vi "CFTS-Get Data Folder.vi"(5 "Drive":string, 7 "Root folder":path, 8 "error in (no error)":errorcluster, 9 "create?":bool, 10 "Number":i32, 11 "Experimenter":string) -> (0 "error out":errorcluster, 2 "Data folder":path)   [LabVIEW 2020]
doc: "Takes an experiment ID (e.g. KEH999) and returns the standard data folder (e.g. C:\\Data\\KEH DATA\\KEH999)"
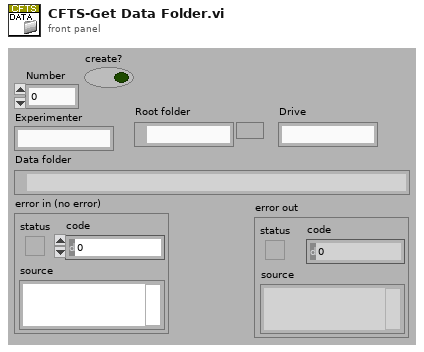
[diagram p1: front panel]
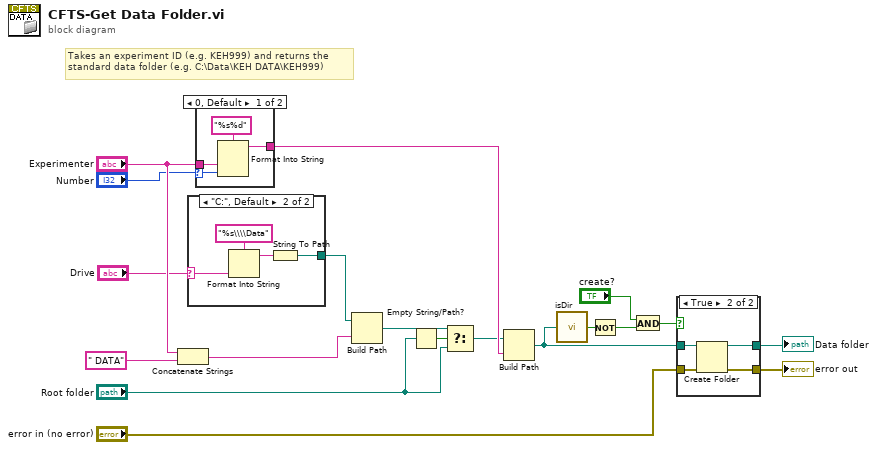
[diagram p0: block diagram]
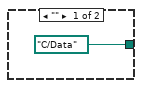
[diagram p2: hidden frame]
diagram:
  # "Takes an experiment ID (e.g. KEH999) and returns the\nstandard data folder (e.g. C:\\Data\\KEH DATA\\KEH999)"
  n1 = Concatenate Strings("Experimenter", " DATA" ("string")) -> (w18:string)
  n2 = case shown="\"C:\", Default" "Drive" {
    selector: "Drive" -> [_ w23]
    tunnel: [path "C:/Data" ("base path") w21] -> w1
    frame "" {
    }
    frame "C:", Default {
      n3 = Format Into String(format string="%s\\\\Data", w23) -> (resulting string=w22:string)  [unwired: 2 in, 1 out]
      n4 = String To Path(string=w22) -> (path=w21:path)
    }
  }
  n5 = case shown="0, Default" "Number" {
    selector: "Number" -> [w26 _]
    tunnel: "Experimenter" -> [w27 w29]
    tunnel: [w25 w29] -> w15
    frame 0, Default {
      n6 = Format Into String(format string="%s%d", w27, w26) -> (resulting string=w25:string)  [unwired: 2 in, 1 out]
    }
    frame -1 {
    }
  }
  n7 = Build Path(base path=w1, name or relative path=w18) -> (appended path=w5:path)
  n8 = Empty String/Path?(string/path="Root folder") -> (empty?=w6:bool)
  n9 = Select(t=w5, s=w6, f="Root folder") -> (s? t:f=w4:path)
  n10 = Build Path(base path=w4, name or relative path=w15) -> (appended path=w14:path)
  n11 = call "isDir.vi"("path"=w14) -> ("is Dir?"=w12:bool)
  n12 = Not(x=w12) -> (.not. x?=w10:bool)
  n13 = And(x="create?", y=w10) -> (x .and. y?=w11:bool)
  n14 = case shown="True" w11 {
    tunnel: w14 -> [w31 w35]
    tunnel: "error in (no error)" -> [w30 w34]
    tunnel: [w31 w33] -> w8
    tunnel: [w30 w32] -> w7
    frame False {
    }
    frame True {
      n15 = Create Folder(path (use dialog)=w35, error in=w34) -> (created path=w33:path, error out=w32:errorcluster)  [unwired: 1 in, 1 out]
    }
  }
  "Data folder" <- w8
  "error out" <- w7
